vi "Destroy.vi"(8 "error in (no error)":errorcluster, 11 "CloneRegRef":refnum<data-value>) -> (0 "error out":errorcluster)   [LabVIEW 2018, in "ModuleAdmin.lvlib" / "CloneRegistration.lvclass"]
uses:
  CloneRegistration.lvclass
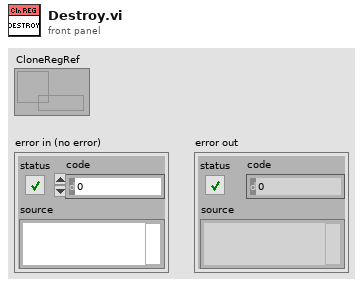
[diagram p1: front panel]
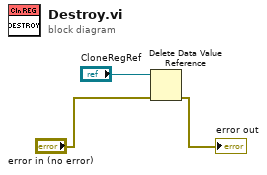
[diagram p0: block diagram]
diagram:
  n1 = Delete Data Value Reference(data value reference="CloneRegRef", error in="error in (no error)") -> (error out=→"error out":errorcluster)  [unwired: 1 out]
